vi "Custom Constant Dialog.vi"(8 "error in":errorcluster) -> (0 "error out":errorcluster, 2 "Cancel Out":bool, 3 "New Constant VI name":string)   [LabVIEW 2020, in "ConstantErrorsMaker.lvlib"]
uses:
  ConstantErrorsMaker.lvlib
  MulticolumListbox.ctl
  Continue.ctl
panel:
  in  "Library Ref":refnum<vi>
  in  "Project Ref":refnum<vi>
  in  "Main App Inst Ref":refnum<vi>
  in  "Project Results":T1 caption="Project Results Table"
  in  "New Constant VI name (do not add --constant.vi)":string
  in  "Continue":T2
  in  "Cancel":bool
  # "TIP: Doble click to open --error.vi Block Diagram"
  # "Constant VIs help manage fixed values efficiently. They work like regular constants but allow centralized editing.\n\nKey Benefits:\n\nSingle Point of Editing: Update the value in one place, and changes apply everywhere.\n\nBetter Maintainability: Clear, modular code makes it easy to find and modify values.\n\nFewer Errors: Reduces typos and inconsistencies across your application."
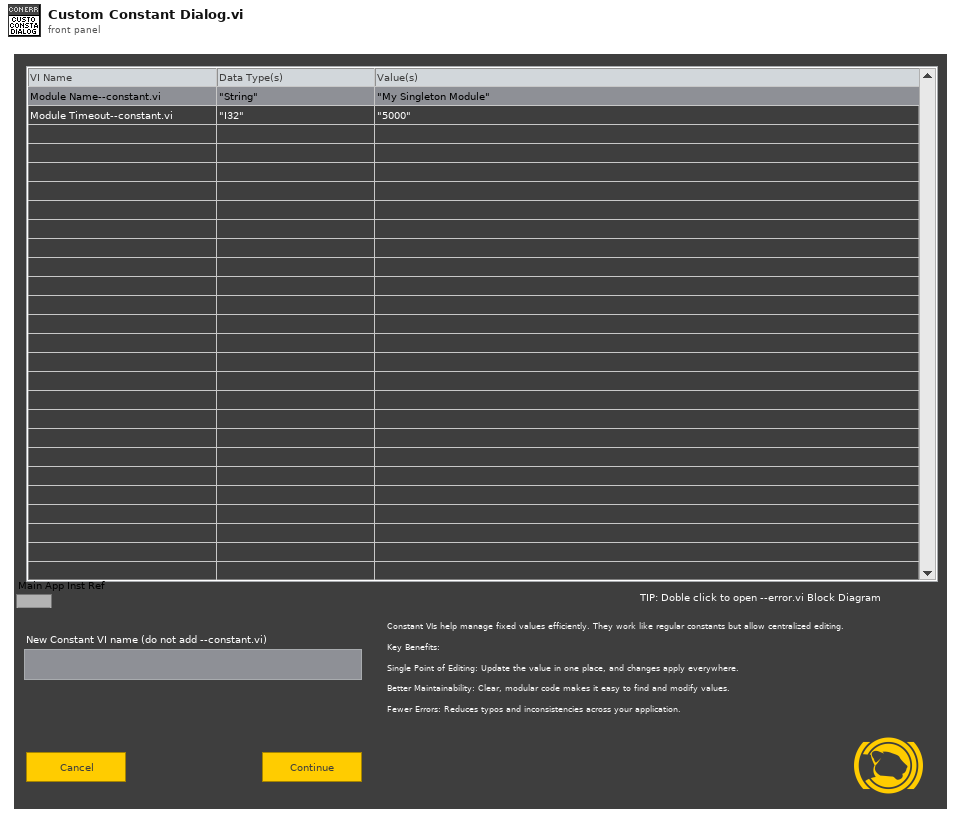
[diagram p1: front panel]
types:
  T1 = typedef "ConstantErrorsMaker.lvlib/MulticolumListbox.ctl" = i32
  T2 = typedef "ConstantErrorsMaker.lvlib/Continue.ctl" = bool
  T3 = typedef "ConstantErrorsMaker.lvlib/Constant Info--cluster.ctl" = cluster{"VI Name":string, "Data Type(s)":string, "Value(s)":string}
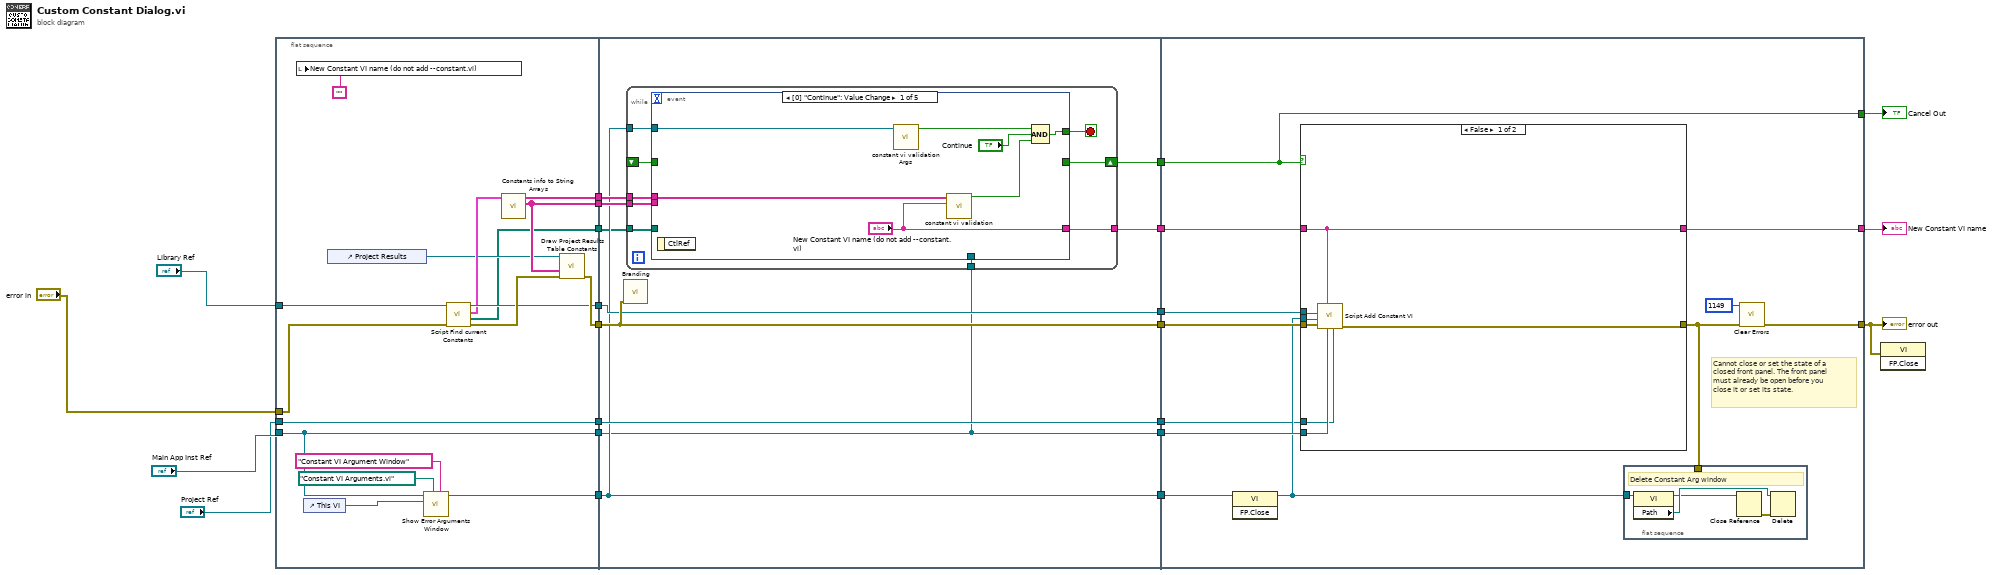
[diagram p0: block diagram]
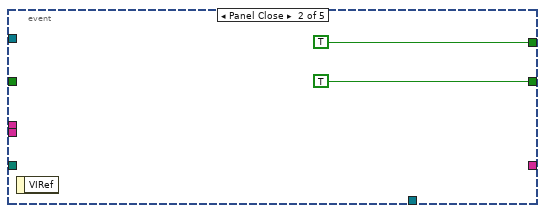
[diagram p2: hidden frame]
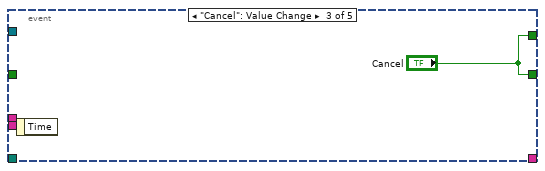
[diagram p3: hidden frame]
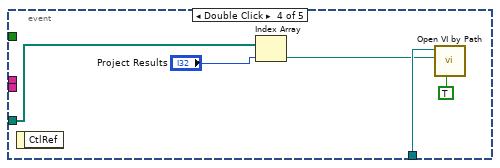
[diagram p4: hidden frame]
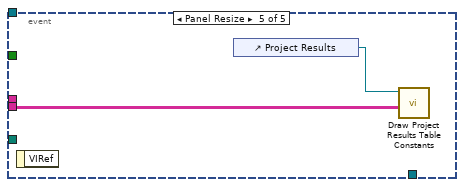
[diagram p5: hidden frame]
diagram:
  n1 = flat-sequence {
    tunnel: "Library Ref" -> [w36]
    tunnel: [w35] -> w16
    tunnel: [w33] -> w14
    tunnel: "Main App Inst Ref" -> [w30]
    tunnel: [w30] -> w13
    tunnel: [w27] -> w10
    tunnel: "Project Ref" -> [w27]
    tunnel: [w26] -> w6
    tunnel: [w25] -> w5
    tunnel: [w38] -> w21
    tunnel: "error in" -> [w37]
    tunnel: [w23] -> w4
    tunnel: [w49] -> w22
    tunnel: [w46] -> w18
    tunnel: [w48] -> w17
    tunnel: w16 -> [w48]
    tunnel: [w42] -> w15
    tunnel: w14 -> [w42]
    tunnel: w13 -> [w40]
    tunnel: [w40] -> w12
    tunnel: [w47] -> w11
    tunnel: w10 -> [w45]
    tunnel: [w45] -> w9
    tunnel: w6 -> [w44]
    tunnel: w5 -> [w43]
    tunnel: w21 -> [w49]
    tunnel: w4 -> [w41]
    tunnel: [w87] -> w19
    tunnel: w22 -> [w85]
    tunnel: w18 -> [w76]
    tunnel: w17 -> [w84]
    tunnel: w15 -> [w83]
    tunnel: w12 -> [w82]
    tunnel: w11 -> [w81]
    tunnel: w9 -> [w78]
    tunnel: [w77] -> w8
    tunnel: [w76] -> w7
    frame #0 {
      n2 = local write "New Constant VI name (do not add --constant.vi)"("") -> ()
      n3 = control-ref of="This VI"() -> (w34:refnum<vi>)
      n4 = control-ref of="Project Results"() -> (w24:refnum<vi>)
      n5 = call "Show Error Arguments Window.vi"("Title"="Constant VI Argument Window", "Path"=path "Constant VI Arguments.vi", "Calling VI Ref"=w34, "App Instance"=w30) -> ("Error Arguments Window Ref"=w33:refnum<vi>)  [unwired: 6 in, 1 out]
      n6 = call "Script Find current Constants.vi"("error in"=w37, "Library in"=w36) -> ("error out"=w39:errorcluster, "All Constant VIS"=w23:path[], "Constants Info"=w28:T3[], "Library out"=w35:refnum<vi>)  [unwired: 6 in]
      n7 = call "Constants info to String Arrays.vi"("Constants Info"=w28) -> ("Constant Info Results Str"=w26:string[][], "VI Names"=w25:string[])  [unwired: 9 in]
      n8 = call "Draw Project Results Table Constants.vi"("error in"=w39, "Constant Results"=w26, "Project Results Ref"=w24) -> ("error out"=w38:errorcluster)  [unwired: 8 in]
    }
    frame #1 {
      n9 = call "Branding.vi"("error in"=w49) -> ()  [unwired: 11 in]
      n10 = while {
        tunnel: w42 -> [w56]
        shift-right: [w57] -> w46
        shift-left: _ -> [w55]
        tunnel: [w54] -> w47
        tunnel: w44 -> [w53]
        tunnel: w43 -> [w52]
        tunnel: w41 -> [w51]
        tunnel: w40 -> [w50]
        stop <- w58 stop-if-true
        n11 = event shown="[0] \"Continue\": Value Change" {
          selector: _ -> [_ _ _ _ _]
          dyn-events: _ -> [_ _ _ _ _]
          timeout: _ -> [_ _ _ _ _]
          tunnel: [w65 TRUE ("Cancel") "Cancel" _ _] -> w58
          tunnel: [_ TRUE ("Cancel") "Cancel" _ _] -> w57
          tunnel: w56 -> [w60 _ _ _ _]
          tunnel: w55 -> [_ _ _ _ _]
          tunnel: ["New Constant VI name (do not add --constant.vi)" _ _ _ _] -> w54
          tunnel: w52 -> [w59 _ _ _ _]
          tunnel: w53 -> [_ _ _ _ w75]
          tunnel: w51 -> [_ _ _ w72 _]
          tunnel: w50 -> [_ _ _ w73 _]
          event Value Change {
            n12 = event-data() -> ()  [unwired: 1 in, 1 out]
            n13 = call "constant vi validation Args.vi"("Constant Argument Window"=w60) -> ("Proceed with Scripting"=w63:bool)  [unwired: 10 in]
            n14 = call "constant vi validation.vi"("New Constant vi name"="New Constant VI name (do not add --constant.vi)", "Constant VI List"=w59) -> ("Proceed with Scripting"=w62:bool)  [unwired: 9 in]
            n15 = Compound Arithmetic op=AND(w63, "Continue", w62) -> (w65:T2)
          }
          event Panel Close {
            n16 = event-data() -> ()  [unwired: 1 in, 1 out]
          }
          event "Cancel": Value Change {
            n17 = event-data() -> ()  [unwired: 1 in, 1 out]
          }
          event Double Click {
            n18 = event-data() -> ()  [unwired: 1 in, 1 out]
            n19 = Index Array(array=w72, index="Project Results") -> (element=w70:path)
            n20 = call "Open VI by Path.vi"("Block Diagram?"=TRUE, "VI Path"=w70, "Application in"=w73) -> ()  [unwired: 8 in, 1 out]
          }
          event Panel Resize {
            n21 = event-data() -> ()  [unwired: 1 in, 1 out]
            n22 = control-ref of="Project Results"() -> (w74:refnum<vi>)
            n23 = call "Draw Project Results Table Constants.vi"("Constant Results"=w75, "Project Results Ref"=w74) -> ()  [unwired: 9 in, 1 out]
          }
        }
      }
    }
    frame #2 {
      # "Cannot close or set the state of a closed front panel. The front panel must already be open before you close it or set its state."
      n24 = invoke class="VI" method="FP.Close"(reference=w83) -> (reference out=w79:refnum<vi>)  [unwired: 2 in, 2 out]
      n25 = case shown="False" w76 {
        tunnel: [w97 w100] -> w86
        tunnel: w85 -> [w98 w100]
        tunnel: w84 -> [w95 _]
        tunnel: w79 -> [w96 _]
        tunnel: w82 -> [w94 _]
        tunnel: w81 -> [w92 w99]
        tunnel: w78 -> [w93 _]
        tunnel: [w92 w99] -> w77
        frame False {
          n26 = call "Script Add Constant VI.vi"("Project Ref"=w93, "App Ref"=w94, "Constant VI Name"=w92, "error in"=w98, "Constant VI Args"=w96, "Library Reference"=w95) -> ("error out"=w97:errorcluster)  [unwired: 5 in]
        }
        frame True {
        }
      }
      n27 = flat-sequence {
        tunnel: w79 -> [w90]
        tunnel: w86 -> [_]
        frame #0 {
          # "Delete Constant Arg window"
          n28 = property class="VI"(reference=w90) -> (reference out=w88:refnum<vi>, "Path"=w89:path)  [unwired: 1 in, 1 out]
          n29 = Close Reference(reference=w88) -> (error out=w91:errorcluster)  [unwired: 1 in]
          n30 = Delete(path (use dialog)=w89, error in=w91) -> ()  [unwired: 3 in, 3 out]
        }
      }
      n31 = call <vilib>:"Clear Errors.vi"("error in (no error)"=w86, "specific error code to clear (0: all)"=1149) -> ("error out"=w87:errorcluster)  [unwired: 4 in, 1 out]
    }
  }
  n32 = invoke class="VI" method="FP.Close"(error in=w19) -> ()  [unwired: 2 in, 3 out]
  "error out" <- w19
  "New Constant VI name" <- w8
  "Cancel Out" <- w7
